vi "Wait-C.vi"(11 "Params":string[][](array[string])) -> ()   [LabVIEW 2020]
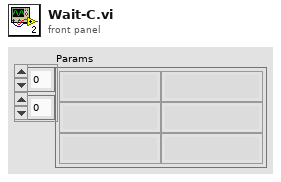
[diagram p1: front panel]
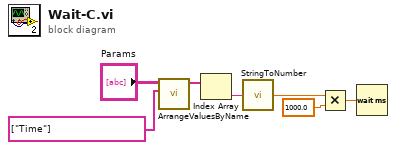
[diagram p0: block diagram]
diagram:
  n1 = call "ArrangeValuesByName.vi"("Names"=string[] ["Time"], "Names/Values in"="Params") -> ("Values Out"=w2:string[])  [unwired: 9 in]
  n2 = Index Array(array=w2) -> (element=w1:string)  [unwired: 1 in]
  n3 = call "StringToNumber.vi"("String"=w1) -> ("Output"=w7:dbl)
  n4 = Multiply(x=w7, y=1000.0) -> (x*y=w5:dbl)
  n5 = Wait (ms)(milliseconds to wait=w5) -> ()  [unwired: 1 out]
